vi "convert code to command.vi"(10 "code":i32) -> (1 "axis number":u8, 2 "command":T1)   [LabVIEW 2010]
uses:
  FPGA scanInfo/scan message.ctl
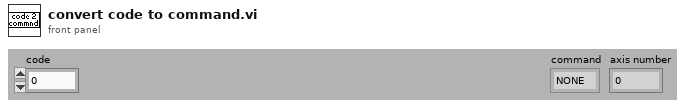
[diagram p1: front panel]
types:
  T1 = typedef "scan message.ctl" = enum8{"NONE", "VOLUME START", "LINE START", "LINE START TRACKING", "XKALMAN", "YKALMAN", "ZKALMAN"}
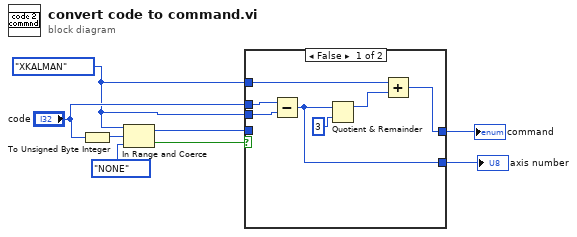
[diagram p0: block diagram]
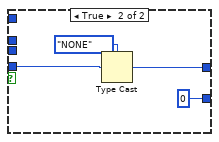
[diagram p2: hidden frame]
diagram:
  w1 = scan_message."XKALMAN" ("Enum")
  n1 = To Unsigned Byte Integer(number="code") -> (unsigned 8bit integer=w8:u8)
  n2 = In Range and Coerce(upper limit=w1, x=w8, lower limit=scan_message."NONE" ("Enum")) -> (coerced(x)=w5:u8, In Range?=w6:bool)
  n3 = case shown="False" w6 {
    tunnel: w5 -> [_ w18]
    tunnel: [w10 w17] -> w4
    tunnel: [w9 u8 0] -> w3
    tunnel: "code" -> [w15 _]
    tunnel: w1 -> [w14 _]
    tunnel: w1 -> [w11 _]
    frame False {
      n4 = Subtract(x=w15, y=w14) -> (x-y=w9:i32)
      n5 = Quotient & Remainder(x=w9, y=3) -> (x-y*floor(x/y)=w12:i32)  [unwired: 1 out]
      n6 = Add(x=w11, y=w12) -> (x+y=w10:i32)
    }
    frame True {
      n7 = Type Cast(type=scan_message."NONE" ("Enum"), x=w18) -> (*(type *) &x=w17:T1)
    }
  }
  "command" <- w4
  "axis number" <- w3
